vi "Read TEC SP.vi"(8 "error in (no error)":errorcluster, 11 "Set TEC SP MSG in":refnum<class "Set TEC SP MSG.lvclass">) -> (0 "error out":errorcluster, 2 "TEC SP":sgl[](array[numeric]), 3 "Set TEC SP MSG out":refnum<class "Set TEC SP MSG.lvclass">)   [LabVIEW 2014, in "Set TEC SP MSG.lvclass"]
uses:
  Set TEC SP MSG.lvclass
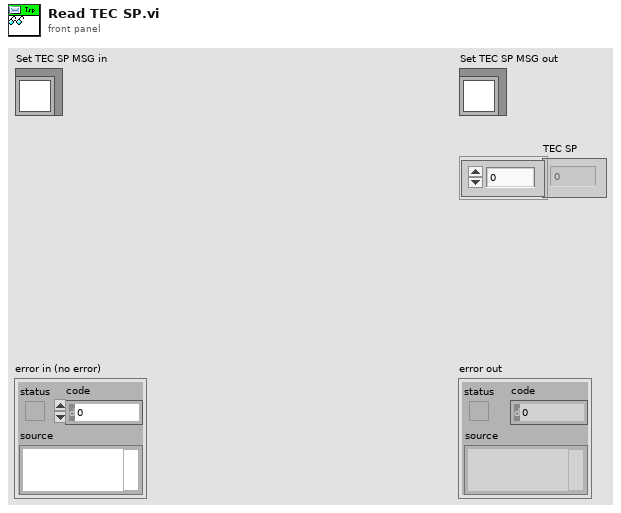
[diagram p1: front panel]
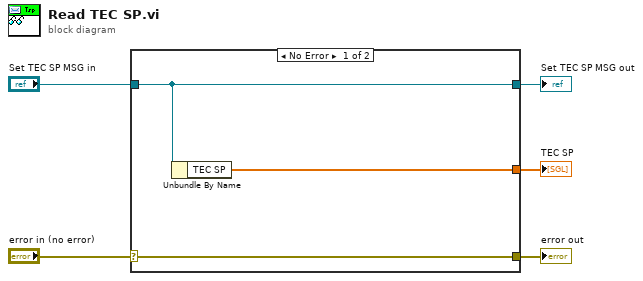
[diagram p0: block diagram]
diagram:
  n1 = case shown="No Error" "error in (no error)" {
    selector: "error in (no error)" -> [w8 w9]
    tunnel: [w8 w9] -> w4
    tunnel: [w7 w10] -> w2
    tunnel: "Set TEC SP MSG in" -> [w7 w10]
    tunnel: [w6 _] -> w1
    frame No Error {
      n2 = Unbundle By Name(w7) -> ("TEC SP"=w6:sgl[])
    }
    frame Error {
    }
  }
  "error out" <- w4
  "Set TEC SP MSG out" <- w2
  "TEC SP" <- w1
